vi "DSF.Memory.Transfer.Set ID.vi"(8 "error in (no error)":errorcluster, 10 "id":i32, 11 "Transfer in":refnum<class "DSF.Memory.Transfer.lvclass">) -> (0 "error out":errorcluster, 3 "Transfer out":refnum<class "DSF.Memory.Transfer.lvclass">)   [LabVIEW 2016, in "DSF.Memory.lvlib" / "DSF.Memory.Transfer.lvclass"]
uses:
  DSF.Memory.Transfer.lvclass
  DSF.Memory.Transfer.lvclass/DSF.Memory.Transfer.ctl
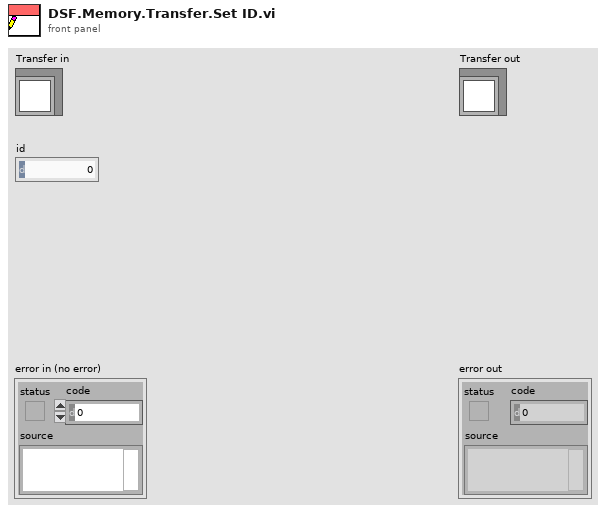
[diagram p1: front panel]
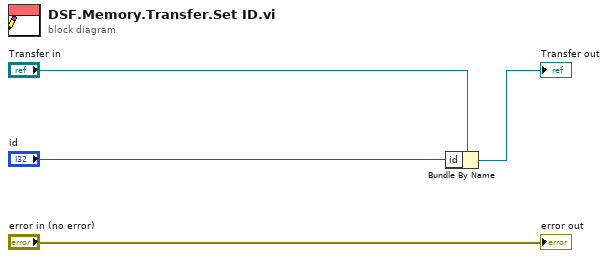
[diagram p0: block diagram]
diagram:
  n1 = Bundle By Name(cluster="Transfer in", "id"="id") -> (→"Transfer out":refnum<class "DSF.Memory.Transfer.lvclass">)
  "error out" <- "error in (no error)"
